vi "Connect.vi"(0 "reference in":refnum<class "Redis.lvclass">, 11 "Error In":errorcluster) -> (4 "reference out":refnum<class "Redis.lvclass">, 8 "Connected?":bool, 15 "Error Out":errorcluster)   [LabVIEW 2020, in "Redis.lvclass"]
uses:
  Redis.lvclass
  ReplyDataTypeEnum.ctl
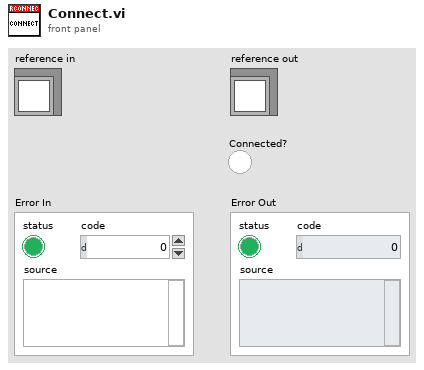
[diagram p1: front panel]
types:
  T1 = typedef "Redis.lvclass/ReplyDataTypeEnum.ctl" = enum16{"None", "Error", "Status", "Nil", "Integer", "String", "Multibulk"}
  T2 = typedef "Redis.lvclass/RedisDataType.ctl" = cluster{"Reply Type":T1, "Integer":i64, "String":string, "Multibulk":variant[], "StringData":string[]}
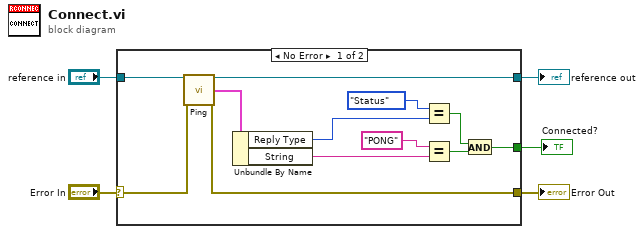
[diagram p0: block diagram]
diagram:
  n1 = case shown="No Error" "Error In" {
    selector: "Error In" -> [w7 w19]
    tunnel: [w6 w19] -> w4
    tunnel: [w11 w18] -> w2
    tunnel: "reference in" -> [w10 w18]
    tunnel: [w12 _] -> w1
    frame No Error {
      n2 = call "Ping.vi"("reference in"=w10, "Error In"=w7) -> ("reference out"=w11:refnum<class "Redis.lvclass">, "Data"=w9:T2, "Error Out"=w6:errorcluster)  [unwired: 11 in]
      n3 = Unbundle By Name(w9) -> ("Reply Type"=w13:T1, "String"=w14:string)
      n4 = Equal?(x=ReplyDataTypeEnum."Status", y=w13) -> (x = y?=w17:bool)
      n5 = Equal?(x="PONG", y=w14) -> (x = y?=w16:bool)
      n6 = And(x=w17, y=w16) -> (x .and. y?=w12:bool)
    }
    frame Error {
    }
  }
  "Error Out" <- w4
  "reference out" <- w2
  "Connected?" <- w1
